vi "Open Net Use.vi"(7 "Login Credentials":T1, 8 "error in (no error)":errorcluster, 10 "Drive Letter (Y)":string="Y", 11 "Net Use Path":path=path "\\\\samba\\val_framework/Staging/VI Packages") -> (0 "error IO":errorcluster, 2 "Net Use Drive Letter":string, 3 "Net Use Connection Path":path)   [LabVIEW 2017, in "G3_Build Process File Utilities.lvlib"]
uses:
  G3_Build Process File Utilities.lvlib
  Net Use Login Credentials.ctl
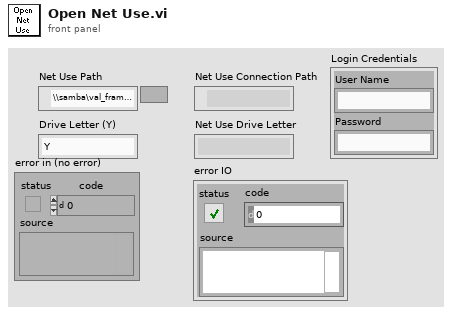
[diagram p1: front panel]
types:
  T1 = typedef "G3_Build Process File Utilities.lvlib/Net Use Login Credentials.ctl" = cluster{"User Name":string, "Password":string}
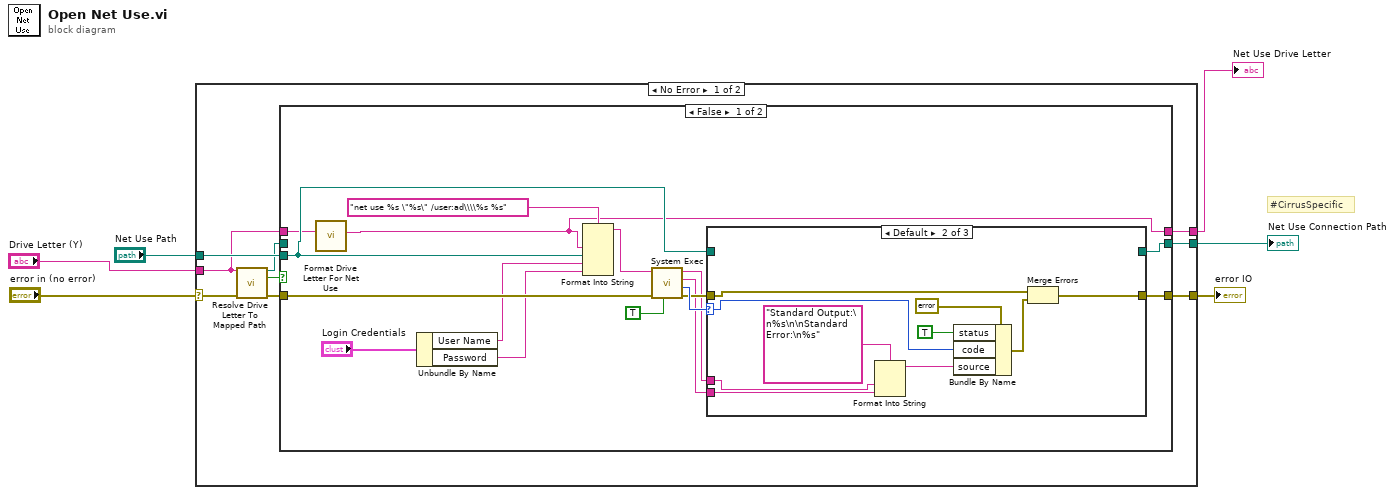
[diagram p0: block diagram]
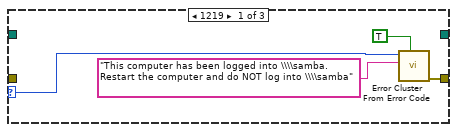
[diagram p2: hidden frame]
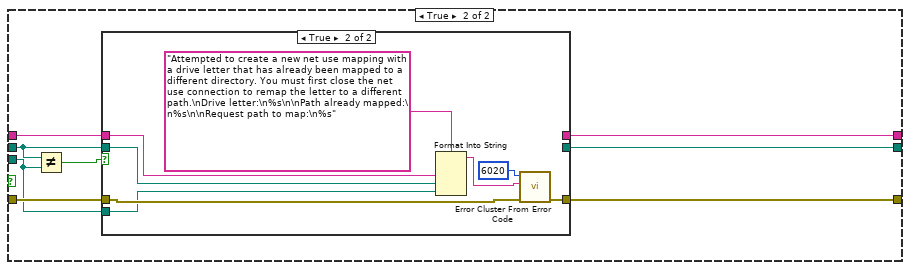
[diagram p4: hidden frame]
diagram:
  # "#CirrusSpecific"
  n1 = case shown="No Error" "error in (no error)" {
    selector: "error in (no error)" -> [w11 w67]
    tunnel: "Net Use Path" -> [w15 _]
    tunnel: [w14 _] -> w5
    tunnel: [w13 w67] -> w4
    tunnel: "Drive Letter (Y)" -> [w12 _]
    tunnel: [w7 _] -> w1
    frame No Error {
      n2 = call "Resolve Drive Letter To Mapped Path.vi"("Drive Letter"=w12, "error in (no error)"=w11) -> ("Mapped Path"=w10:path, "Found"=w8:bool, "error out"=w9:errorcluster)  [unwired: 11 in]
      n3 = case shown="False" w8 {
        tunnel: w15 -> [w22 w52]
        tunnel: [w21 w55] -> w14
        tunnel: [w25 w53] -> w13
        tunnel: w12 -> [w20 w49]
        tunnel: w10 -> [_ w51]
        tunnel: w9 -> [w23 w54]
        tunnel: [w19 w48] -> w7
        frame False {
          n4 = call "Format Drive Letter For Net Use.vi"("Drive Letter"=w20) -> ("String"=w19:string)  [unwired: 10 in]
          n5 = Unbundle By Name("Login Credentials") -> ("User Name"=w17:string, "Password"=w16:string)
          n6 = Format Into String(format string="net use %s \"%s\" /user:ad\\\\%s %s", w19, w22, w17, w16) -> (resulting string=w31:string)  [unwired: 2 in, 1 out]
          n7 = call <vilib>:"System Exec.vi"("run minimized? (F)"=TRUE, "error in (no error)"=w23, "command line"=w31) -> ("error out"=w28:errorcluster, "return code"=w29:i32, "standard error"=w26:string, "standard output"=w27:string)  [unwired: 5 in]
          n8 = case shown="Default" w29 {
            selector: w29 -> [w34 w43 _]
            tunnel: w28 -> [_ w38 w47]
            tunnel: w27 -> [_ w41 _]
            tunnel: w26 -> [_ w40 _]
            tunnel: [w35 w36 w47] -> w25
            tunnel: w22 -> [_ _ w46]
            tunnel: [_ _ w46] -> w21
            frame 1219 {
              n9 = call <vilib>:"Error Cluster From Error Code.vi"("show call chain? (False)"=TRUE, "error message (\"\")"="This computer has been logged into \\\\samba. Restart the computer and do NOT log into \\\\samba" ("error message (\"\")"), "error code (0)"=w34) -> ("error out"=w35:errorcluster)  [unwired: 6 in]
            }
            frame Default {
              n10 = Format Into String(format string="Standard Output:\n%s\n\nStandard Error:\n%s", w41, w40) -> (resulting string=w39:string)  [unwired: 2 in, 1 out]
              n11 = Bundle By Name(cluster=errorcluster {"status"=FALSE, "code"=0, "source"=""} ("error out"), "status"=TRUE, "code"=w43, "source"=w39) -> (w37:errorcluster)
              n12 = Merge Errors(w38, w37) -> (w36:errorcluster)
            }
            frame 0 {
            }
          }
        }
        frame True {
          n13 = Not Equal?(x=w51, y=w52) -> (x != y?=w50:bool)
          n14 = case shown="True" w50 {
            tunnel: [w58 _] -> w55
            tunnel: w51 -> [w58 w60]
            tunnel: w54 -> [w57 w66]
            tunnel: [w57 w65] -> w53
            tunnel: w49 -> [w56 w61]
            tunnel: w52 -> [_ w59]
            tunnel: [w56 _] -> w48
            frame False {
            }
            frame True {
              n15 = Format Into String(format string="Attempted to create a new net use mapping with a drive letter that has already been mapped to a different directory. You must first close the net use connection to remap the letter to a different path.\nDrive letter:\n%s\n\nPath already mapped:\n%s\n\nRequest path to map:\n%s", w61, w60, w59) -> (resulting string=w63:string)  [unwired: 2 in, 1 out]
              n16 = call <vilib>:"Error Cluster From Error Code.vi"("error in (no error)"=w66, "error message (\"\")"=w63, "error code (0)"=6020) -> ("error out"=w65:errorcluster)  [unwired: 6 in]
            }
          }
        }
      }
    }
    frame Error {
    }
  }
  "Net Use Connection Path" <- w5
  "Net Use Drive Letter" <- w1
  "error IO" <- w4
